vi "IsSpeedingUp.vi"(11 "Input":dbl) -> (3 "Speeding Up?":bool)   [LabVIEW 2016]
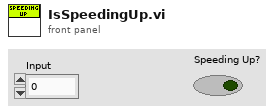
[diagram p1: front panel]
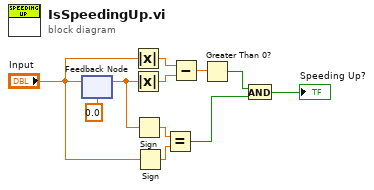
[diagram p0: block diagram]
diagram:
  n1 = feedback-in #1("Input") -> ()
  n2 = feedback #1(0.0 ("Input")) -> (w7:dbl)
  n3 = Absolute Value(x="Input") -> (abs(x)=w9:dbl)
  n4 = Absolute Value(x=w7) -> (abs(x)=w10:dbl)
  n5 = Sign(1:w7) -> (0:w6:dbl)
  n6 = Sign(1:"Input") -> (0:w5:dbl)
  n7 = Equal?(x=w6, y=w5) -> (x = y?=w4:bool)
  n8 = Subtract(x=w9, y=w10) -> (x-y=w3:dbl)
  n9 = Greater Than 0?(x=w3) -> (x > 0?=w2:bool)
  n10 = And(x=w2, y=w4) -> (x .and. y?=→"Speeding Up?":bool)
